vi "SetExposure.vi"(8 "error in (no error)":errorcluster, 10 "value":dbl, 11 "Photometrics Cam v2 in":refnum<class "Photometrics_CH-250_Cam.lvclass">) -> (0 "error out":errorcluster, 3 "Photometrics Cam v2 out":refnum<class "Photometrics_CH-250_Cam.lvclass">)   [LabVIEW 2013, in "Photometrics_CH-250_Cam.lvclass"]
uses:
  Photometrics_CH-250_Cam.lvclass
  CameraSessionClass/CS250-CameraHardwareClass.lvclass
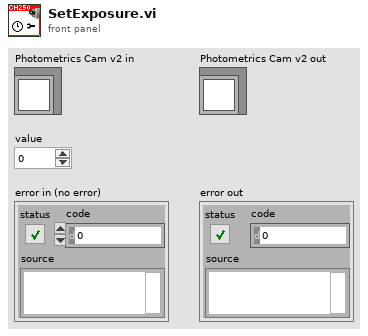
[diagram p1: front panel]
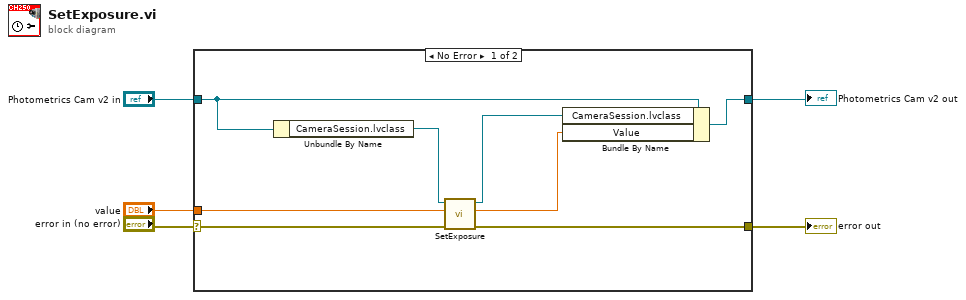
[diagram p0: block diagram]
diagram:
  n1 = case shown="No Error" "error in (no error)" {
    selector: "error in (no error)" -> [w6 w15]
    tunnel: [w13 w15] -> w5
    tunnel: "value" -> [w10 _]
    tunnel: "Photometrics Cam v2 in" -> [w8 w14]
    tunnel: [w7 w14] -> w2
    frame No Error {
      n2 = Unbundle By Name(w8) -> ("CameraSession.lvclass"=w9:refnum<class "CS250-CameraHardwareClass.lvclass">)
      n3 = call-dynamic "SetExposure.vi"("error in (no error)"=w6, "Exposure"=w10, "CameraSession  in"=w9) -> ("error out"=w13:errorcluster, "ExposureReadback(Sec)"=w11:dbl, "CameraSession out"=w12:refnum<class "CS250-CameraHardwareClass.lvclass">)  [unwired: 5 in, 1 out]
      n4 = Bundle By Name(cluster=w8, "CameraSession.lvclass"=w12, "Value"=w11) -> (w7:refnum<class "Photometrics_CH-250_Cam.lvclass">)
    }
    frame Error {
    }
  }
  "error out" <- w5
  "Photometrics Cam v2 out" <- w2
